vi "AutoDriveStraightthenBalance.vi"(8 "error in (no error)":errorcluster, 9 "TimeOut (s)":dbl, 10 "MaxSpeed (ft/s)":dbl, 11 "Dist (ft)":dbl) -> (0 "error out":errorcluster)   [LabVIEW 2020]
doc: "Wrapper class for drive straight"
uses:
  <vilib>/Utility/semaphor.llb/Obtain Semaphore Reference.vi
  <vilib>/Rock Robotics/WPI/ThirdParty/JAS_Junk/TrajLib/Timer_Reset.vi
  <vilib>/Rock Robotics/WPI/ThirdParty/JAS_Junk/TrajLib/Trajectory_Library.lvlib
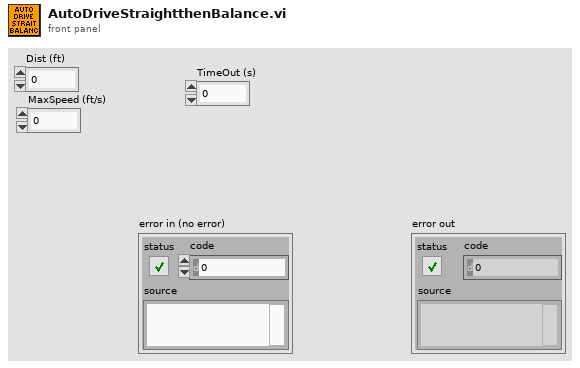
[diagram p1: front panel]
types:
  T1 = typedef "Trajectory_Library.lvlib/TIMER.ctl" = cluster{"StartTime":dbl, "Accumulated TIme":dbl, "Running":bool, "semaphore":T2}
  T2 = typedef "Semaphore RefNum" = refnum<k1>
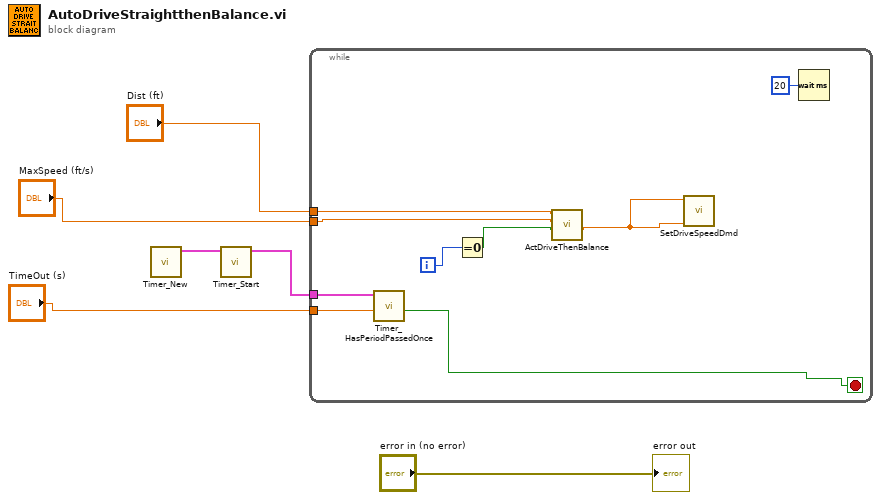
[diagram p0: block diagram]
diagram:
  n1 = call <vilib>:"Timer_New.vi"() -> ("TIMER"=w3:T1)  [unwired: 11 in]
  n2 = call <vilib>:"Timer_Start.vi"("in Timer"=w3) -> ("out Timer"=w2:T1)  [unwired: 10 in]
  n3 = while {
    tunnel: "Dist (ft)" -> [w11]
    tunnel: "MaxSpeed (ft/s)" -> [w10]
    tunnel: w2 -> [w14]
    tunnel: "TimeOut (s)" -> [w13]
    i -> [w15]
    stop <- w8 stop-if-true
    n4 = call <vilib>:"Timer_HasPeriodPassedOnce.vi"("Period"=w13, "in Timer"=w14) -> ("Expired"=w8:bool)  [unwired: 7 in, 2 out]
    n5 = Equal To 0?(x=w15) -> (x = 0?=w9:bool)
    n6 = call "ActDriveThenBalance.vi"("FirstTime"=w9, "MaxSpeed (ft/s)"=w10, "Dist (ft)"=w11) -> ("XSpeedDemand"=w7:dbl)  [unwired: 7 in, 1 out]
    n7 = call "SetDriveSpeedDmd.vi"("LeftSpeedInput"=w7, "RightSpeedInput"=w7) -> ()  [unwired: 10 in]
    n8 = Wait (ms)(milliseconds to wait=u32 20) -> ()  [unwired: 1 out]
  }
  "error out" <- "error in (no error)"
